vi "AddSpaces.vi"(7 "Text.Selection":T1, 8 "Add Spaces?":bool, 11 "String in":refnum<vi>) -> (1 "Cursor":cluster{u32, u32}, 3 "String out":refnum<vi>)   [LabVIEW 2020]
uses:
  <vilib>/Utility/miscctls.llb/LVSelectionTypeDef.ctl
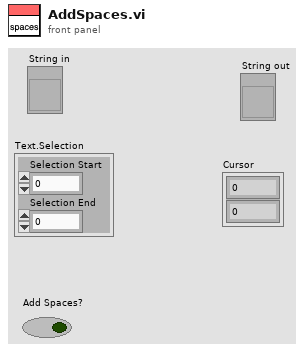
[diagram p1: front panel]
types:
  T1 = typedef "LVSelectionTypeDef.ctl" = cluster{"Selection Start":u32, "Selection End":u32}
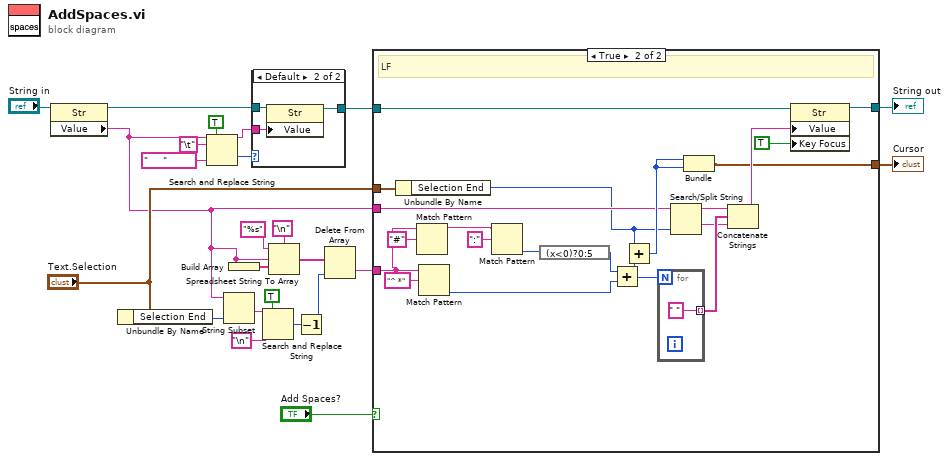
[diagram p0: block diagram]
diagram:
  n1 = property on="Property Node" class="Str"(reference="String in") -> (reference out=w6:refnum<vi>, "Value"=w3:string)  [unwired: 1 in, 1 out]
  n2 = Unbundle By Name("Text.Selection") -> ("Selection End"=w20:u32)
  n3 = Search and Replace String(replace all?=TRUE ("replace all? (F)"), input string=w3, search string="\t", replace string="     " ("replace string (\"\")")) -> (result string=w9:string, number of replacements=w10:i32)  [unwired: 4 in, 2 out]
  n4 = String Subset(string=w3, length (rest)=w20) -> (substring=w19:string)  [unwired: 1 in]
  n5 = Build Array(w3) -> (w5:string[])
  n6 = case shown="Default" w10 {
    tunnel: w6 -> [w25 w28]
    tunnel: [w25 w27] -> w8
    tunnel: w9 -> [_ w26]
    frame 0 {
    }
    frame Default {
      n7 = property on="Property Node" class="Str"(reference=w28, "Value"=w26) -> (reference out=w27:refnum<vi>)  [unwired: 1 in, 1 out]
    }
  }
  n8 = Search and Replace String(replace all?=TRUE ("replace all? (F)"), input string=w19, search string="\n") -> (number of replacements=w16:i32)  [unwired: 5 in, 3 out]
  n9 = Spreadsheet String To Array(delimiter (Tab)="\n", format string="%s", spreadsheet string=w3, array type (2D Dbl)=w5) -> (array=w4:string[])
  n10 = Decrement(x=w16) -> (x-1=w15:i32)
  n11 = Delete From Array(array=w4, index=w15) -> (deleted portion=w24:string)  [unwired: 1 in, 1 out]
  n12 = case shown="True" "Add Spaces?" {
    tunnel: w24 -> [_ w50]
    tunnel: w3 -> [_ w35]
    tunnel: w8 -> [w29 w42]
    tunnel: [w29 w41] -> w23
    tunnel: "Text.Selection" -> [w30 w38]
    tunnel: [w30 w31] -> w14
    frame False {
    }
    frame True {
      # "LF"
      n13 = Unbundle By Name(w38) -> ("Selection End"=w34:u32)
      n14 = Match Pattern(string=w50, regular expression="#") -> (before substring=w47:string)  [unwired: 1 in, 3 out]
      n15 = Match Pattern(string=w50, regular expression="^ *") -> (offset past match=w44:i32)  [unwired: 1 in, 3 out]
      n16 = Match Pattern(string=w47, regular expression=":") -> (offset past match=w46:i32)  [unwired: 1 in, 3 out]
      n17 = expression code="(x<0)?0:5"(w46) -> (w45:i32)
      n18 = Add(x=w45, y=w44) -> (x+y=w37:i32)
      n19 = Add(x=w34, y=w37) -> (x+y=w36:u32)
      n20 = for {
        N: w37 -> [_]
        tunnel: [" " ("regular expression")] -> w43 mode=indexing
      }
      n21 = Search/Split String(string=w35, offset (0)=w34) -> (substring before match=w33:string, match + rest of string=w32:string)  [unwired: 1 in, 1 out]
      n22 = Bundle(w36, w36) -> (w31:cluster{u32, u32})  [unwired: 1 in]
      n23 = Concatenate Strings(w33, w43, w32) -> (w40:string)
      n24 = property class="Str"(reference=w42, "Value"=w40, "Key Focus"=TRUE) -> (reference out=w41:refnum<vi>)  [unwired: 1 in, 1 out]
    }
  }
  "String out" <- w23
  "Cursor" <- w14
